vi "Constructor.vi"(5 "TimeZoneInfoId (Local)":string="Local", 7 "GenerationTime (Now)":timestamp, 8 "error in":errorcluster) -> (0 "error out":errorcluster, 3 "Datawarehouse":refnum<class "Datawarehouse.lvclass">)   [LabVIEW 2021, in "ProligentXMLGenerator.lvlib" / "Datawarehouse.lvclass"]
doc: "Creates a ProligentCanonicalFile in memory"
uses:
  Datawarehouse.lvclass
  Datawarehouse.lvclass/Datawarehouse.ctl
  <vilib>/xml/NI_XML.lvlib
  Failure/Defect/Defect.lvclass
  Data.ctl
  Base/DateTime/DateTime.lvclass
  Base/NonEmptyString_2000/NonEmptyString_2000.lvclass
  Base/NonEmptyString_448/NonEmptyString_448.lvclass
  ProcessRun/ProcessRun.lvclass
  ProligentXMLGenerator.lvlib
  ProductUnit/ProductUnit.lvclass
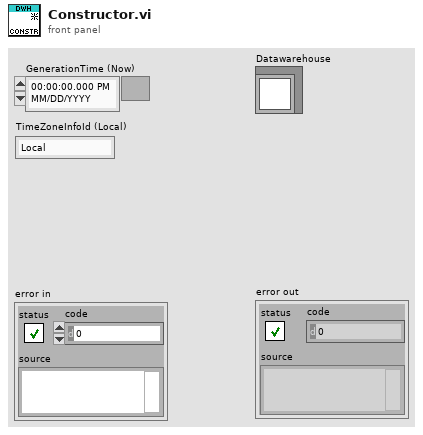
[diagram p1: front panel]
types:
  T1 = typedef "ProligentXMLGenerator.lvlib/Datawarehouse.lvclass/Data.ctl" = cluster{"DestinationFolder":path, "BaseFileName":string, "Document":refnum<k20>, "Defects":refnum<class "Defect.lvclass">[], "TopProcessRuns":refnum<class "ProcessRun.lvclass">[], "ProductUnits":refnum<class "ProductUnit.lvclass">[], "GenerationTime":refnum<class "DateTime.lvclass">, "DataSourceFingerprint":refnum<class "NonEmptyString_448.lvclass">, "IntegrationMetaData":refnum<class "NonEmptyString_2000.lvclass">, "TimeZoneInfoId":string}
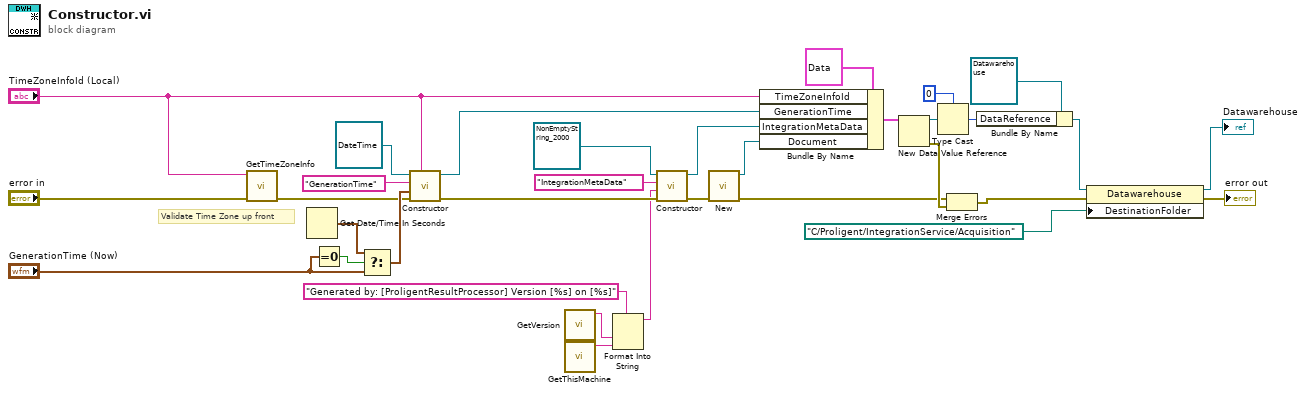
[diagram p0: block diagram]
diagram:
  # "Validate Time Zone up front"
  n1 = call "GetTimeZoneInfo.vi"("error in"="error in", "TimeZoneInfoId"="TimeZoneInfoId (Local)") -> ("error out"=w2:errorcluster)  [unwired: 7 in, 2 out]
  n2 = Get Date/Time In Seconds() -> (seconds since 1Jan1904=w7:timestamp)
  n3 = Equal To 0?(x="GenerationTime (Now)") -> (x = 0?=w8:bool)
  n4 = Select(t=w7, s=w8, f="GenerationTime (Now)") -> (s? t:f=w5:timestamp)
  n5 = call-dynamic "Constructor.vi"("TimeZoneInfoId"="TimeZoneInfoId (Local)", "error in"=w2, "Value"=w5, "Name"="GenerationTime", "DateTime in"=refnum<class "DateTime.lvclass"> refnum) -> ("error out"=w17:errorcluster, "DateTime out"=w23:refnum<class "DateTime.lvclass">)  [unwired: 5 in]
  n6 = call "GetVersion.vi"() -> ("Version"=w15:string)  [unwired: 11 in]
  n7 = call "GetThisMachine.vi"() -> ("ThisMachine"=w4:string)  [unwired: 11 in]
  n8 = Format Into String(format string="Generated by: [ProligentResultProcessor] Version [%s] on [%s]" ("regular expression"), w15, w4) -> (resulting string=w13:string)  [unwired: 2 in, 1 out]
  n9 = call-dynamic "Constructor.vi"("error in"=w17, "Value"=w13, "Name"="IntegrationMetaData" ("time format string (%c)"), "String in"=refnum<class "NonEmptyString_2000.lvclass"> refnum ("ProligentCanonicalFile:NonEmptyString_2000")) -> ("error out"=w19:errorcluster, "String out"=w18:refnum<class "NonEmptyString_2000.lvclass">)  [unwired: 6 in]
  n10 = call <vilib>:"New.vi"("error in (no error)"=w19) -> ("error out"=w26:errorcluster, "DOM document out"=w27:refnum<k20>)  [unwired: 7 out]
  n11 = Bundle By Name(cluster=T1 {"DestinationFolder"=path "", "BaseFileName"="", "Document"=refnum, "Defects"=[], "TopProcessRuns"=[], "ProductUnits"=[], "GenerationTime"=refnum, "DataSourceFingerprint"=refnum, "IntegrationMetaData"=refnum, "TimeZoneInfoId"=""} ("Data"), "TimeZoneInfoId"="TimeZoneInfoId (Local)", "GenerationTime"=w23, "IntegrationMetaData"=w18, "Document"=w27) -> (w22:T1)
  n12 = New Data Value Reference(data value=w22) -> (data value reference=w29:refnum<data-value>, error out=w32:errorcluster)  [unwired: 1 in]
  n13 = Type Cast(type=u64 0, x=w29) -> (*(type *) &x=w31:u64)
  n14 = Merge Errors(w26, w32) -> (w33:errorcluster)
  n15 = Bundle By Name(cluster=refnum<class "Datawarehouse.lvclass"> refnum ("Datawarehouse"), "DataReference"=w31) -> (w11:refnum<class "Datawarehouse.lvclass">)
  n16 = property class="Datawarehouse"(reference=w11, error in=w33, "DestinationFolder"=path "C:/Proligent/IntegrationService/Acquisition") -> (reference out=→"Datawarehouse":refnum<class "Datawarehouse.lvclass">, error out=→"error out":errorcluster)
